vi "Fluke 189 Data Logger.vi"() -> ()   [LabVIEW 2017]
doc: "This VI can be used to setup the fl18x multimeter and read a measurement.\n\nNote:\n(1) Prior to calling this function, the rotary switch must be set manually to the desired measurement."
uses:
  <vilib>/Platform/TimedLoop/XDataNode/timing_clust.ctl
  <vilib>/Platform/TimedLoop/XDataNode/nitl_modes.ctl
  <vilib>/Platform/TimedLoop/XDataNode/wakeup.ctl
  <vilib>/platform/TimedLoop/XDataNode/XDataNode.xnode
  <instrlib>/Fluke 18X Series/Fluke 189 Series.lvlib
  <vilib>/Platform/TimedLoop/XDataNode/XDNodeRunTimeDep.lvlib
panel:
  in  "Relative Reset":bool
  in  "MinMaxAvg Reset":bool
  out "Waveform Chart":dbl(graph)
  in  "stop":bool
  in  "VISA resource name":refnum<visa-resource-name>
  in  "Function (Exit Rel)":enum16{"Exit Rel", "Relative", "% Relative"}(ring)
  in  "Range (5V)":T1(ring)
  in  "Function (Auto)":enum16{"Auto Range", "Manual Range"}(ring)
  in  "Type (0:Normal Min/Max Mode)":T2(ring)
  in  "Function (0:Exit Min/Max Mode)":T3(ring)
  out "Units":T4(ring)
  out "Measurement":dbl caption="Measurement:" format="%.3f"
  out "Error out":errorcluster {"code" format="%x"}
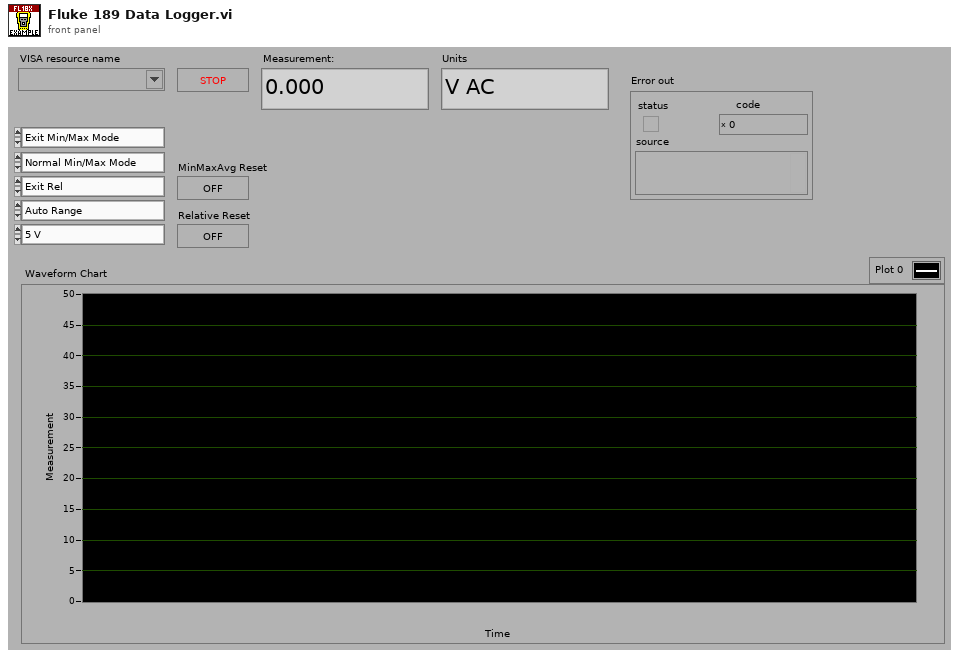
[diagram p1: front panel]
types:
  T1 = enum16{"5 V", "50 V", "500 V", "1000 V", "50 mV", "500 mV", "5000 mV", "500 Ohms", "5 kOhms", "50 kOhms", "500 kOhms", "5 MOhms", "30 MOhms", "500 MOhms", "1 uF", "10 uF", "100 uF", "1 mF", "10 mF", "50 mF", "5 A", "10 A", "50 mA", "500 mA", "500 uA", "5000 uA"}
  T2 = enum16{"Normal Min/Max Mode", "Fast Min/Max Mode"}
  T3 = enum16{"Exit Min/Max Mode", "Display Minimum Value", "Display Maximum Value", "Display Average Value"}
  T4 = enum16{"V AC", "mV AC", "V DC", "mV DC", "V AC+DC", "mV AC+DC", "Ohms", "kOhms", "MOhms", "nS", "nFarads", "uFarads", "mFarads", "A AC", "mA AC", "uA AC", "A DC", "mA DC", "uA DC", "A AC+DC", "mA AC+DC", "uA AC+DC", "Deg C", "Deg F", "dBm", "dBV", "Hz", "%", "ms"}
  T5 = typedef "XDNodeRunTimeDep.lvlib/timing_clust.ctl" = cluster{"Expected End [f-1]":u64, "Actual End [f-1]":u64, "Finished Late? [f-1]":bool, "Expected End [i-1]":u64, "Actual End [i-1]":u64, "Finished Late? [i-1]":bool, "Expected Start [i]":u64, "Actual Start [i]":u64, "Expected Start [f]":u64, "Actual Start [f]":u64, "Source Name":string, "Structure Name":string, "Period":i64, "Deadline":i64, "Offset":i64, "Start":i64, "Priority":i32, "Timeout":i32, "Mode":T6, "Wakeup Reason":T7, "Error":errorcluster, "Source Type":string, "Secondary Source Type":string, "Global End Time":u64, "Global Start Time":u64, "Frame Duration":u64, "Iteration Duration":u64, "Assigned CPU":i32, "I/O Scan Engine Mode":u32}
  T6 = typedef "XDNodeRunTimeDep.lvlib/nitl_modes.ctl" = enum32{"No Change", "Process missed periods, maintain original phase", "Discard missed periods, maintain original phase", "Process missed periods, ignore original phase", "Discard missed periods, ignore original phase"}
  T7 = typedef "XDNodeRunTimeDep.lvlib/wakeup.ctl" = enum32{"Normal", "Aborted", "Asynchronous wakeup", "Timing source error", "Timed loop error", "Timeout"}
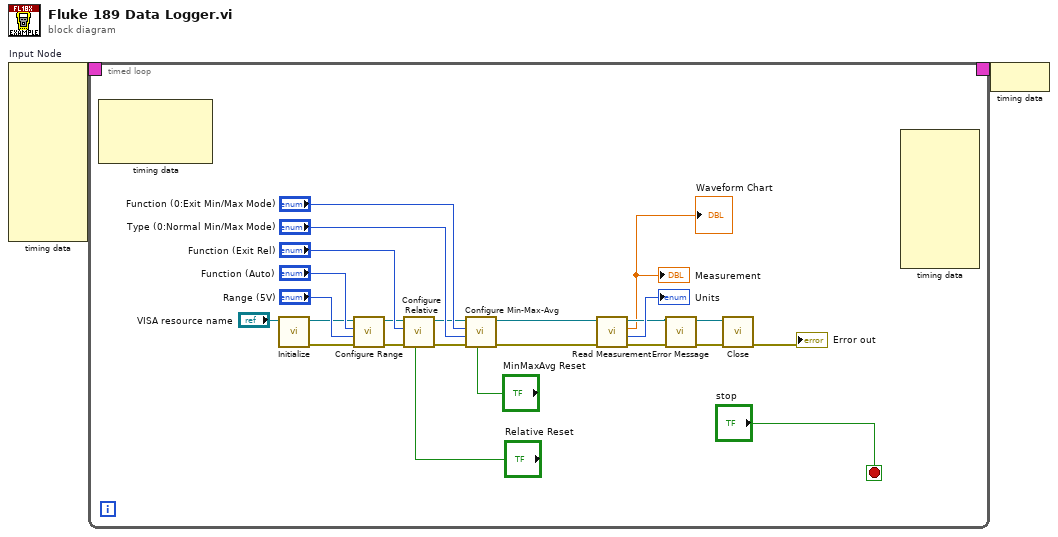
[diagram p0: block diagram]
diagram:
  n1 = node-c288 "Input Node"() -> (w2:T5)  [unwired: 10 in]
  n2 = timed-loop {
    timing: w2 -> [_]
    timing-out: [_] -> w1
    stop <- "stop" stop-if-true
    n3 = node-c288() -> ()  [unwired: 1 in, 3 out]
    n4 = call <instrlib>:"Initialize.vi"("VISA resource name"="VISA resource name") -> ("error out"=w12:errorcluster, "VISA resource name out"=w13:refnum<visa-resource-name>)  [unwired: 9 in]
    n5 = call <instrlib>:"Configure Range.vi"("error in (no error)"=w12, "Range (5V)"="Range (5V)", "Function (Exit Manual)"="Function (Auto)", "VISA resource name"=w13) -> ("error out"=w17:errorcluster, "VISA resource name out"=w20:refnum<visa-resource-name>)  [unwired: 6 in]
    n6 = call <instrlib>:"Configure Relative.vi"("Reset"="Relative Reset", "error in (no error)"=w17, "Function (Exit Rel)"="Function (Exit Rel)", "VISA resource name"=w20) -> ("error out"=w16:errorcluster, "VISA resource name out"=w19:refnum<visa-resource-name>)  [unwired: 6 in]
    n7 = call <instrlib>:"Configure Min-Max-Avg.vi"("Reset"="MinMaxAvg Reset", "error in (no error)"=w16, "Type (0:Normal Min/Max Mode)"="Type (0:Normal Min/Max Mode)", "Function (0:Exit Min/Max Mode)"="Function (0:Exit Min/Max Mode)", "VISA resource name"=w19) -> ("error out"=w5:errorcluster, "VISA resource name out"=w18:refnum<visa-resource-name>)  [unwired: 5 in]
    n8 = call <instrlib>:"Read Measurement.vi"("error in (no error)"=w5, "VISA resource name"=w18) -> ("error out"=w9:errorcluster, "Units"=→"Units":T4, "Measurement"=→"Measurement" →"Waveform Chart":dbl, "VISA resource name out"=w10:refnum<visa-resource-name>)  [unwired: 6 in]
    n9 = call <instrlib>:"Error Message.vi"("error in (no error)"=w9, "VISA resource name"=w10) -> ("error out"=w8:errorcluster, "VISA resource name out"=w6:refnum<visa-resource-name>)  [unwired: 5 in, 3 out]
    n10 = call <instrlib>:"Close.vi"("error in (no error)"=w8, "VISA resource name"=w6) -> ("error out"=→"Error out":errorcluster)  [unwired: 9 in]
    n11 = node-c288() -> ()  [unwired: 8 in, 1 out]
  }
  n12 = node-c288(w1) -> ()
